vi "全局 总氮.vi"() -> ()   [LabVIEW 2016]
panel:
  in  "总氮":string[][](array[string])
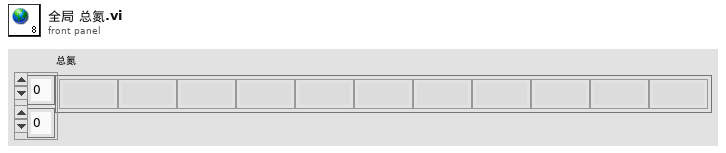
[diagram p1: front panel]
diagram:
